vi "Konstanten zum Tabellen initialisieren.vi"() -> (4 "Anzahl Gaskomponenten":i32, 8 "Anzahl Tabellenzeilen":i32, 15 "Anzahl Tabellenspalten":i32)   [LabVIEW 2020, in "Linearisierung v2.lvlib"]
uses:
  Linearisierung v2.lvlib
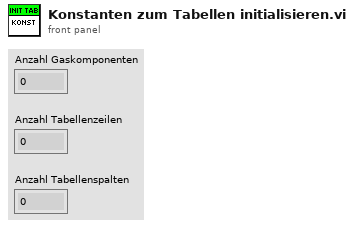
[diagram p1: front panel]
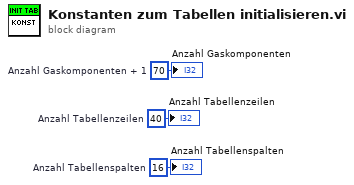
[diagram p0: block diagram]
diagram:
  w1 = 40  # Anzahl Tabellenzeilen
  w2 = 16  # Anzahl Tabellenspalten
  w3 = 70  # Anzahl Gaskomponenten + 1
  "Anzahl Gaskomponenten" <- w3
  "Anzahl Tabellenspalten" <- w2
  "Anzahl Tabellenzeilen" <- w1
